vi "Launcher.vi"   [LabVIEW 2023]
uses:
  Plant/Plant/Plant.lvclass
  C:/Program Files (x86)/National Instruments/LabVIEW 2023/vi.lib/ActorFramework/Actor/Actor.lvclass
  Plant/Plant Messages/Write Ambient Msg/Write Ambient Msg.lvclass/Write Ambient Msg.ctl
  <vilib>/ActorFramework/Message Enqueuer/Message Enqueuer.lvclass/Message Enqueuer.ctl
  Plant/Plant Messages/Write PID gains Msg/Write PID gains Msg.lvclass/Write PID gains Msg.ctl
  Plant/Plant Messages/Write Target Msg/Write Target Msg.lvclass/Write Target Msg.ctl
  <vilib>/ActorFramework/Message Enqueuer/Enqueue.vi
  Plant/Plant Messages/Write Ambient Msg/Write Ambient Msg.lvclass
  C:/Program Files (x86)/National Instruments/LabVIEW 2023/vi.lib/ActorFramework/Message/Message.lvclass
  Plant/Plant Messages/Write PID gains Msg/Write PID gains Msg.lvclass
  Plant/Plant Messages/Write Target Msg/Write Target Msg.lvclass
  <vilib>/ActorFramework/Stop Msg/Stop Msg.lvclass
  <vilib>/ActorFramework/Message Priority Queue/Priority Enqueue.vi
  <vilib>/ActorFramework/Actor/Actor.lvclass
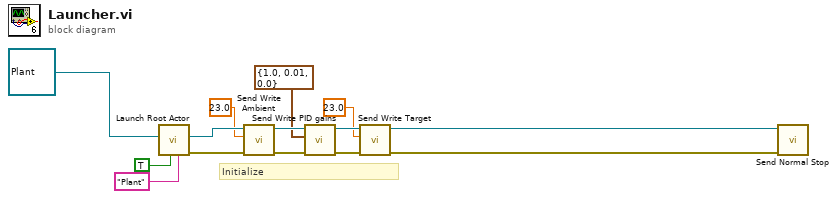
[diagram p0: block diagram]
diagram:
  # "Initialize"
  n1 = call <vilib>:"Launch Root Actor.vi"("Debug Alias"="Plant", "Open Actor Core front panel? (F)"=TRUE, "Actor"=refnum<class "Plant.lvclass"> refnum ("Plant.lvlib:Plant.lvclass")) -> ("error out"=w13:errorcluster, "Actor's Enqueuer"=w12:refnum<class "Message Enqueuer.lvclass">)  [unwired: 7 in]
  n2 = call "Send Write Ambient.vi"("error in (no error)"=w13, "Ambient"=23.0, "Message Enqueuer"=w12) -> ("error out"=w8:errorcluster, "Message Enqueuer out"=w11:refnum<class "Message Enqueuer.lvclass">)  [unwired: 7 in]
  n3 = call "Send Write PID gains.vi"("error in (no error)"=w8, "PID gains"=cluster{"P":dbl, "I":dbl, "D":dbl} {"P"=1.0, "I"=0.01, "D"=0.0}, "Message Enqueuer"=w11) -> ("error out"=w9:errorcluster, "Message Enqueuer out"=w10:refnum<class "Message Enqueuer.lvclass">)  [unwired: 7 in]
  n4 = call "Send Write Target.vi"("error in (no error)"=w9, "Target"=23.0, "Message Enqueuer"=w10) -> ("error out"=w3:errorcluster, "Message Enqueuer out"=w2:refnum<class "Message Enqueuer.lvclass">)  [unwired: 7 in]
  n5 = call <vilib>:"Send Normal Stop.vi"("error in (no error)"=w3, "Message Enqueuer"=w2) -> ()  [unwired: 9 in, 1 out]
